vi "loop.vi"() -> ()   [LabVIEW 2017]
panel:
  out "Iteration":i32
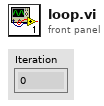
[diagram p1: front panel]
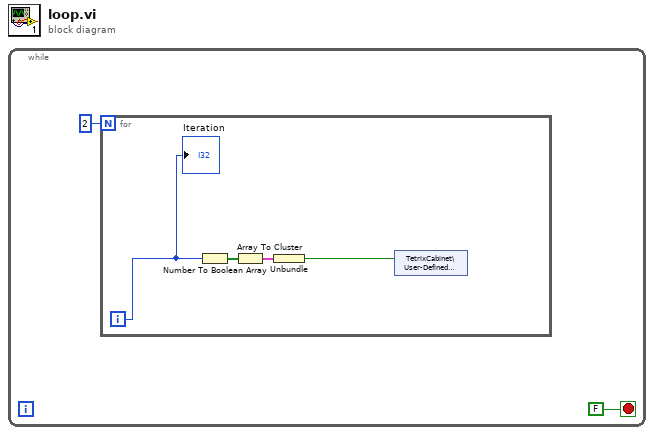
[diagram p0: block diagram]
diagram:
  n1 = while {
    stop <- FALSE stop-if-true
    n2 = for {
      N: 2 -> [_]
      i -> [w4]
      n3 = Number To Boolean Array(number=w4) -> (Boolean array=w6:bool[])
      n4 = Array To Cluster(array=w6) -> (cluster=w5:cluster{"Boolean array[0]":bool})
      n5 = Unbundle(w5) -> ("Boolean array[0]"=w3:bool)
      n6 = shared-variable "TetrixCabinet\\User-Defined Variables\\Input"(w3) -> ()  [unwired: 1 in, 1 out]
      "Iteration" <- w4
    }
  }
